vi "PipBoy_ConfigurePipBoyInterface.vi"(8 "error in (no error)":errorcluster, 10 "PageNum":i32, 11 "PipBoyData":T1) -> (0 "error out":errorcluster)   [LabVIEW 2014]
uses:
  ctls/PipBoy_PipBoyData.ctl
  ctls/PipBoy_ProcComm.ctl
  System.Windows.Forms
  ctls/PipBoy_PipBoyCommand.ctl
  ctls/PipBoy_Message.ctl
  modules/support/Message Queue/All Message Queues.ctl
  modules/support/Message Queue/Message Cluster.ctl
  ctls/PipBoy_FileConf.ctl
  ctls/PipBoy_PicComm.ctl
  ctls/PipBoy_GeneralParams.ctl
  ctls/PipBoy_Pages.ctl
  modules/support/Message Queue/Message Queue.lvlib
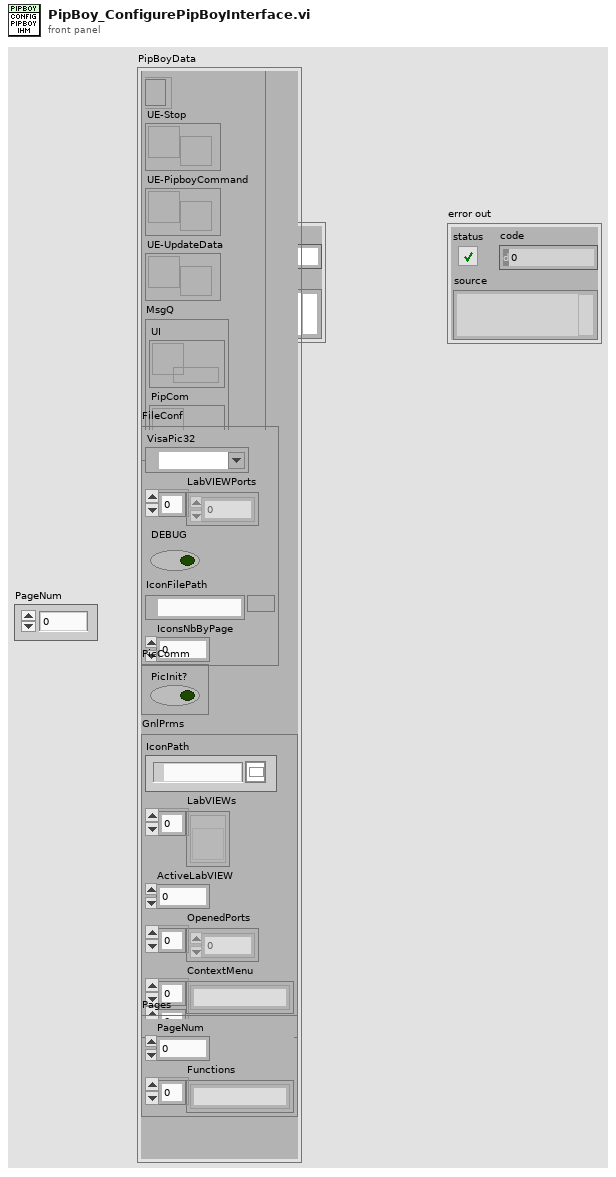
[diagram p1: front panel]
types:
  T1 = typedef "PipBoy_PipBoyData.ctl" = cluster{"ProcComm":T2, "FileConf":T4, "PicComm":T5, "GnlPrms":T6, "Pages":T7}
  T2 = typedef "PipBoy_ProcComm.ctl" = cluster{"NotifyIconRef":refnum<k24>, "UE-Stop":refnum<user-event>, "UE-PipboyCommand":refnum<user-event>, "UE-UpdateData":refnum<user-event>, "MsgQ":T3}
  T3 = typedef "Message Queue.lvlib/All Message Queues.ctl" = cluster{"UI":refnum<queue>, "PipCom":refnum<queue>}
  T4 = typedef "PipBoy_FileConf.ctl" = cluster{"VisaPic32":refnum<visa-resource-name>, "LabVIEWPorts":u16[], "DEBUG":bool, "IconFilePath":path, "IconsNbByPage":i32}
  T5 = typedef "PipBoy_PicComm.ctl" = cluster{"PicInit?":bool}
  T6 = typedef "PipBoy_GeneralParams.ctl" = cluster{"IconPath":path, "LabVIEWs":refnum<vi>[], "ActiveLabVIEW":i32, "OpenedPorts":u16[], "ContextMenu":string[][]}
  T7 = typedef "PipBoy_Pages.ctl" = cluster{"PageNum":i32, "Functions":string[]}
  T8 = typedef "imagedata.ctl" = cluster{"image type":i32, "image depth":i32, "image":u8[], "mask":u8[], "colors":u32[], "Rectangle":cluster{"left":i16, "top":i16, "right":i16, "bottom":i16}}
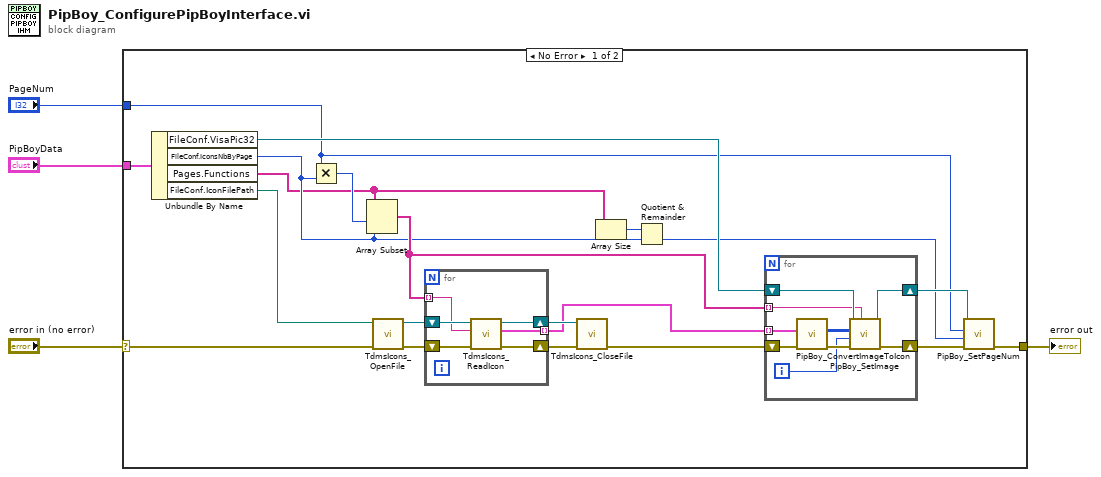
[diagram p0: block diagram]
diagram:
  n1 = case shown="No Error" "error in (no error)" {
    selector: "error in (no error)" -> [w21 w40]
    tunnel: [w8 w40] -> w3
    tunnel: "PipBoyData" -> [w24 _]
    tunnel: "PageNum" -> [w6 _]
    frame No Error {
      n2 = Unbundle By Name(w24) -> ("FileConf.VisaPic32"=w14:refnum<visa-resource-name>, "FileConf.IconsNbByPage"=w11:i32, "Pages.Functions"=w10:string[], "FileConf.IconFilePath"=w22:path)
      n3 = Multiply(x=w6, y=w11) -> (x*y=w23:i32)
      n4 = Array Subset(array=w10, index=w23, length=w11) -> (w12:string[])
      n5 = call "TdmsIcons_OpenFile.vi"("error in (no error)"=w21, "Path"=w22) -> ("error out"=w19:errorcluster, "TdmsOut"=w20:refnum<k34>)  [unwired: 8 in]
      n6 = for {
        tunnel: w12 -> [w36] mode=indexing
        shift-right: [w37] -> w17
        shift-left: w19 -> [w38]
        tunnel: [w35] -> w16 mode=indexing
        shift-right: [w34] -> w18
        shift-left: w20 -> [w39]
        n7 = call "TdmsIcons_ReadIcon.vi"("error in (no error)"=w38, "Function"=w36, "TdmsIn"=w39) -> ("error out"=w37:errorcluster, "Icon"=w35:T8, "TdmsOut"=w34:refnum<k34>)  [unwired: 6 in]
      }
      n8 = call "TdmsIcons_CloseFile.vi"("error in (no error)"=w17, "TdmsIn"=w18) -> ("error out"=w15:errorcluster)  [unwired: 8 in, 1 out]
      n9 = Array Size(array=w10) -> (size(s)=w13:i32)
      n10 = Quotient & Remainder(x=w13, y=w11) -> (floor(x/y)=w5:i32)  [unwired: 1 out]
      n11 = for {
        tunnel: w16 -> [w29] mode=indexing
        shift-right: [w28] -> w9
        shift-left: w15 -> [w33]
        tunnel: w12 -> [w26] mode=indexing
        shift-right: [w25] -> w7
        shift-left: w14 -> [w27]
        i -> [w30]
        n12 = call "PipBoy_ConvertImageToIcon.vi"("error in (no error)"=w33, "Image"=w29) -> ("error out"=w32:errorcluster, "Icon"=w31:u16[][])  [unwired: 8 in]
        n13 = call "PipBoy_SetImage.vi"("Function"=w26, "error in (no error)"=w32, "Image to draw"=w30, "Icon"=w31, "VisaPic32In"=w27) -> ("error out"=w28:errorcluster, "VisaPic32Out"=w25:refnum<visa-resource-name>)  [unwired: 5 in]
      }
      n14 = call "PipBoy_SetPageNum.vi"("error in (no error)"=w9, "PageTot"=w5, "PageNum"=w6, "VisaPic32In"=w7) -> ("error out"=w8:errorcluster)  [unwired: 6 in, 1 out]
    }
    frame Error {
    }
  }
  "error out" <- w3
